vi "XIPIN_DDR3_SDRAM_PHY_IP_1_1.vi"   [LabVIEW 2017]
doc: "PHY for DDR3 interfaces for Ultrascale Architecture\n------------------------------------\n<b>Need License</b> : No"
uses:
  <vilib>/rvi/XilinxIP/XIPIN_XNode/niFpgaXIPIN.xnode
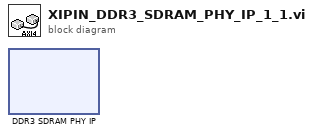
[diagram p0: block diagram]
diagram:
  n1 = xnode ("DDR3 SDRAM PHY IP")() -> ()
